vi "Favorit_Load.vi"(10 "Value":i32, 11 "ItemNames":string[][](array[string])) -> (3 "Array":dbl[](array[numeric]))   [LabVIEW 2015]
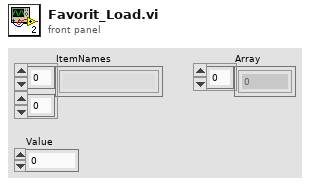
[diagram p1: front panel]
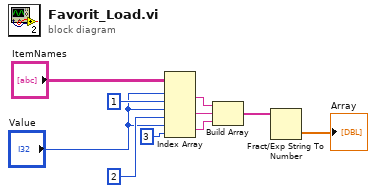
[diagram p0: block diagram]
diagram:
  n1 = Index Array(array="ItemNames", index (row) #1="Value", index (col) #1=1 ("disabled index (col)"), index (row) #2="Value", index (col) #2=2 ("disabled index (col)"), index (row) #3="Value", index (col) #3=3 ("disabled index (col)")) -> (element #1=w6:string, element #2=w7:string, element #3=w8:string)
  n2 = Build Array(w6, w7, w8) -> (w9:string[])
  n3 = Fract/Exp String To Number(string=w9) -> (number=→"Array":dbl[])  [unwired: 3 in, 1 out]
